vi "MB Slave Read Holding Registers (poly).vi"(1 "Starting Address":u16, 2 "Quantity":u16, 5 "error in":errorcluster) -> (15 "Holding Registers":u16[](array[numeric]), 19 "error out":errorcluster)   [LabVIEW 2011]
doc: "Returns the slave holding registers from Starting Address to Starting Address + Quantity."
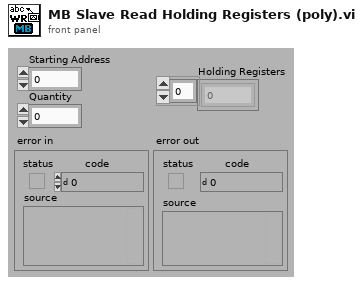
[diagram p1: front panel]
types:
  T1 = enum16{"Discrete Inputs", "Coils", "Input Registers", "Holding Registers"}
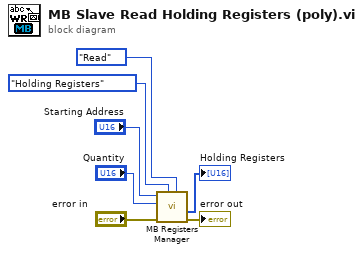
[diagram p0: block diagram]
diagram:
  n1 = call "MB Registers Manager.vi"("Function"=enum16{"Init", "Read", "Write", "Read All"}."Read", "Table"=T1."Holding Registers", "error in (no error)"="error in", "Length"="Quantity", "Start Address"="Starting Address") -> ("error out"=→"error out":errorcluster, "Words out"=→"Holding Registers":u16[])  [unwired: 2 in, 3 out]
